vi "graph_spectrum.vi"(1 "SPECTRUM":dbl[][](array[numeric]), 2 "WAVELENGTH":sgl[](array[numeric])) -> (0 "GRAPHE SPECTRUM":cluster{"WAVELENGTH":dbl[], "SPECTRUM":dbl[]}[](array[cluster]))   [LabVIEW 2018]
panel:
  out "partie supprimée":dbl[][](array[numeric])
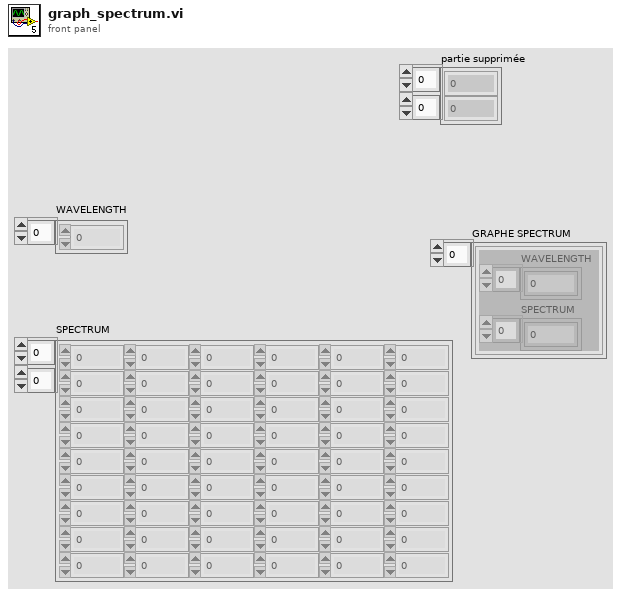
[diagram p1: front panel]
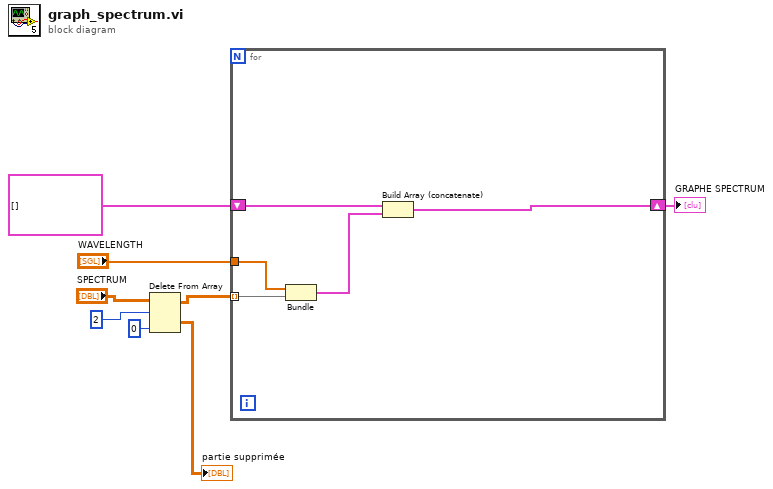
[diagram p0: block diagram]
diagram:
  n1 = Delete From Array(array="SPECTRUM", length=2 ("longueur"), index (col)=0 ("indice désactivé (col)")) -> (deleted portion=→"partie supprimée":dbl[][], array with subset deleted=w2:dbl[][])  [unwired: 1 in]
  n2 = for {
    tunnel: w2 -> [w12] mode=indexing
    tunnel: "WAVELENGTH" -> [w13]
    shift-right: [w10] -> w6
    shift-left: cluster{"WAVELENGTH":dbl[], "SPECTRUM":dbl[]}[] [] -> [w9]
    n3 = Bundle("WAVELENGTH"=w13, "SPECTRUM"=w12) -> (w11:cluster{"WAVELENGTH":sgl[], "SPECTRUM":dbl[]})  [unwired: 1 in]
    n4 = Build Array (concatenate)(w9, w11) -> (w10:cluster{"WAVELENGTH":dbl[], "SPECTRUM":dbl[]}[])
  }
  "GRAPHE SPECTRUM" <- w6
